vi "Create.vi"(0 "Cal Folder":path, 7 "Fs (Hz)":dbl=100000.0) -> (8 "SigMan":refnum<class "SignalManager.lvclass">)   [LabVIEW 2020, in "SignalManager.lvclass"]
uses:
  SignalManager.lvclass
  SignalManager.lvclass/SignalManager.ctl
panel:
  in  "Rig":string
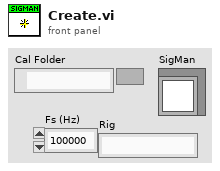
[diagram p1: front panel]
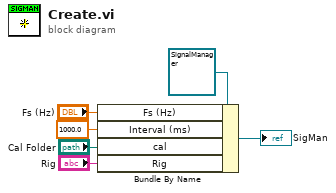
[diagram p0: block diagram]
diagram:
  n1 = Bundle By Name(cluster=refnum<class "SignalManager.lvclass"> refnum ("SigMan"), "Fs (Hz)"="Fs (Hz)", "Interval (ms)"=1000.0 ("Serialized.Interval (ms)"), "cal"="Cal Folder", "Rig"="Rig") -> (→"SigMan":refnum<class "SignalManager.lvclass">)
